vi "Control_BOut.vi"(0 "T-On (s)":dbl, 1 "Estado":bool, 2 "Off Manual":bool, 5 "Error In":errorcluster) -> (14 "Estado_OUT":bool, 19 "Error Out":errorcluster)   [LabVIEW 2013]
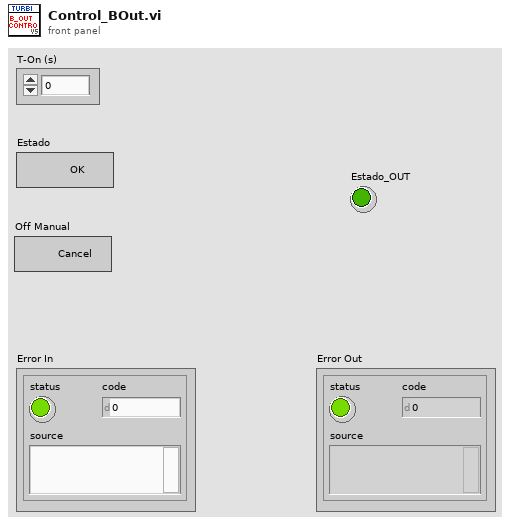
[diagram p1: front panel]
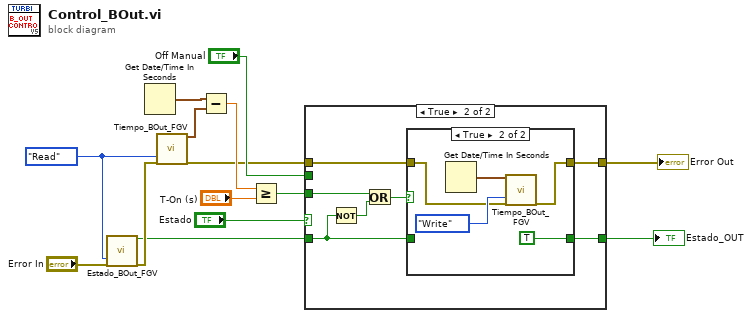
[diagram p0: block diagram]
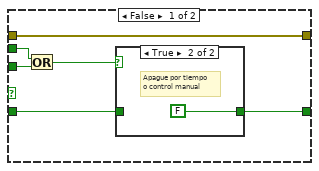
[diagram p2: hidden frame]
diagram:
  w10 = enum16{"Write", "Read"}."Read" ("Opción")
  n1 = call "Estado_BOut_FGV.vi"("Opción"=w10, "Error In"="Error In") -> ("Estado OUT"=w1:bool, "Error Out"=w8:errorcluster)  [unwired: 16 in]
  n2 = Get Date/Time In Seconds() -> (seconds since 1Jan1904=w14:timestamp)
  n3 = call "Tiempo_BOut_FGV.vi"("Opción"=w10, "Error In"=w8) -> ("Tiempo_OUT"=w13:timestamp, "Error Out"=w3:errorcluster)  [unwired: 15 in, 1 out]
  n4 = Subtract(x=w14, y=w13) -> (x-y=w12:dbl)
  n5 = Greater Or Equal?(x=w12, y="T-On (s)") -> (x >= y?=w6:bool)
  n6 = case shown="True" "Estado" {
    tunnel: w6 -> [w20 w29]
    tunnel: "Off Manual" -> [w19 _]
    tunnel: w1 -> [w17 w24]
    tunnel: [w16 w25] -> w4
    tunnel: w3 -> [w15 w27]
    tunnel: [w15 w26] -> w2
    frame False {
      n7 = Or(x=w19, y=w20) -> (x .or. y?=w18:bool)
      n8 = case shown="True" w18 {
        tunnel: [w21 FALSE] -> w16
        tunnel: w17 -> [w21 _]
        frame False {
          # "Mantenga estado"
        }
        frame True {
          # "Apague por tiempo\no control manual"
        }
      }
    }
    frame True {
      n9 = Not(x=w24) -> (.not. x?=w28:bool)
      n10 = Or(x=w29, y=w28) -> (x .or. y?=w23:bool)
      n11 = case shown="True" w23 {
        tunnel: w27 -> [w31 w34]
        tunnel: [w31 w33] -> w26
        tunnel: [w30 TRUE] -> w25
        tunnel: w24 -> [w30 _]
        frame False {
        }
        frame True {
          n12 = Get Date/Time In Seconds() -> (seconds since 1Jan1904=w36:timestamp)
          n13 = call "Tiempo_BOut_FGV.vi"("Tiempo_IN"=w36, "Opción"=enum16{"Write", "Read"}."Write", "Error In"=w34) -> ("Error Out"=w33:errorcluster)  [unwired: 14 in, 2 out]
        }
      }
    }
  }
  "Error Out" <- w2
  "Estado_OUT" <- w4
